vi "Pose_Add.vi"(9 "other TRANSFORM":T4, 11 "in POSE":T1) -> (3 "out POSe":T1)   [LabVIEW 2019, in "PathExecution_Library.lvlib"]
uses:
  PathExecution_Library.lvlib
  POSE.ctl
  TRANSLATION.ctl
  ROTATION.ctl
  TRANSFORM.ctl
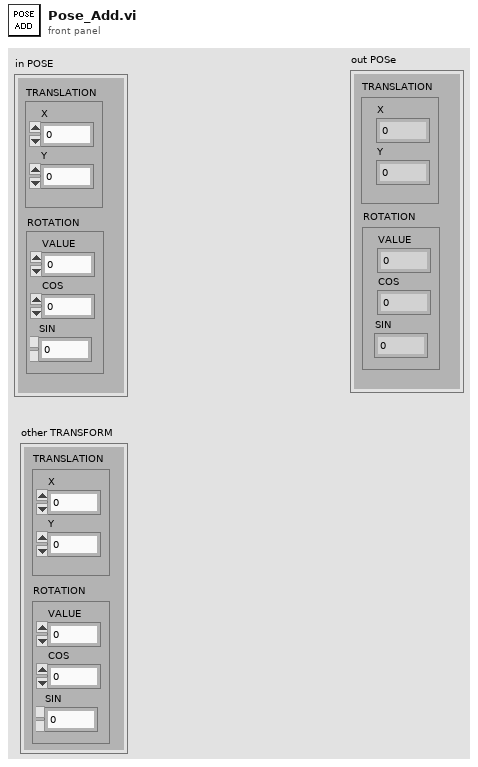
[diagram p1: front panel]
types:
  T1 = typedef "PathExecution_Library.lvlib/POSE.ctl" = cluster{"TRANSLATION":T2, "ROTATION":T3}
  T2 = typedef "PathExecution_Library.lvlib/TRANSLATION.ctl" = cluster{"X":dbl, "Y":dbl}
  T3 = typedef "PathExecution_Library.lvlib/ROTATION.ctl" = cluster{"VALUE":dbl, "COS":dbl, "SIN":dbl}
  T4 = typedef "PathExecution_Library.lvlib/TRANSFORM.ctl" = cluster{"TRANSLATION":T2, "ROTATION":T3}
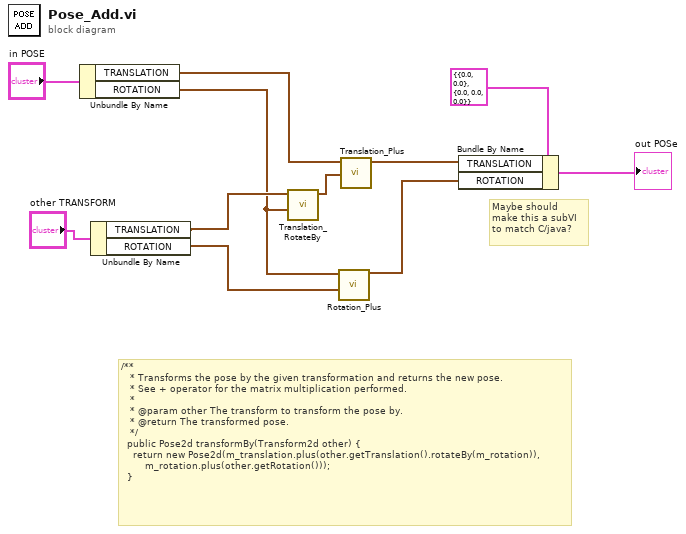
[diagram p0: block diagram]
diagram:
  # "Maybe should\nmake this a subVI \nto match C/java?"
  # "/**\n   * Transforms the pose by the given transformation and returns the new pose.\n   * See + operator for the matrix multiplication performed.\n   *\n   * @param other The transform to transform the pose by.\n   * @return The transformed pose.\n   */\n  public Pose2d transformBy(Transform2d other) {\n    return new Pose2d(m_translation.plus(other.getTranslation().rotateBy(m_rotation)),\n        m_rotation.plus(other.getRotation()));\n  }"
  n1 = Unbundle By Name("in POSE") -> ("TRANSLATION"=w7:T2, "ROTATION"=w3:T3)
  n2 = Unbundle By Name("other TRANSFORM") -> ("TRANSLATION"=w9:T2, "ROTATION"=w2:T3)
  n3 = call "Translation_RotateBy.vi"("other Rotation"=w3, "In Translation"=w9) -> ("Out Translation"=w8:T2)  [unwired: 9 in]
  n4 = call "Rotation_Plus.vi"("other ROTATION"=w2, "in ROTATION"=w3) -> ("out ROTATION"=w1:T3)  [unwired: 9 in]
  n5 = call "Translation_Plus.vi"("other Translation"=w8, "In Translation"=w7) -> ("Out Translation"=w4:T2)  [unwired: 9 in]
  n6 = Bundle By Name(cluster=T1 {"TRANSLATION"={"X"=0.0, "Y"=0.0}, "ROTATION"={"VALUE"=0.0, "COS"=0.0, "SIN"=0.0}} ("sumPOSE"), "TRANSLATION"=w4, "ROTATION"=w1) -> (→"out POSe":T1)
